vi "Scale Module (Main).vi"(7 "Name of Parent Panel":string="Main.vi", 9 "New Center Coords":T1={"Horizontal"=470, "Vertical"=200}, 10 "Config":variant, 11 "Main UI Message Queue":refnum<queue>) -> ()   [LabVIEW 2018, in "Scale Module.lvlib"]
doc: "This Continuous Measurement sample project is based on the Queued Message Handler template.\n\nThe Event Handling Loop generates messages based on user interface actions.\n\nThe Message Handling Loop processes messages generated by the Event Handling Loop, or by other messages. There are also Acquisition and Logging message handling loop subVIs, and a chart updating loop."
uses:
  Scale Module.lvlib
  support/Message Queue/Message Cluster.ctl
  <vilib>/Utility/miscctls.llb/LVPoint32TypeDef.ctl
  controls/UI State.ctl
  Feed Module/Controls/Scale Module State Cluster.ctl
  Feed Module/Controls/Scale Module Config Cluster.ctl
  Feed Module/Controls/Scale Module Settings Cluster.ctl
  Mettler Toledo/Controls/Settings Cluster.ctl
  Feed Module/Controls/Scale Module Display.ctl
  support/Message Queue/Enqueue Message (Single).vi
  support/User Event - Stop/User Event - Stop.lvlib
  support/Message Queue/Message Queue.lvlib
  support/Support Library.lvlib
  Measure Instrument/Scale Module Engine.lvlib
  Mettler Toledo/Mettler Toledo.lvlib
  Scale Settings Dialog.vi
  support/Command Log VIs/Command Logging.lvlib
  Report Generation/Report Generation.lvlib
panel:
  in  "Settings Button":bool
  out "Display Cluster":cluster{"User Name":string, "g":dbl} {"g" format="%#_5f"}
  out "H/W":dbl
  out "Original Height":u32
  out "Original Width":u32
  out "ScanCode":i16
  out "Log File path":path
  out "Status":string
  in  "Exit":bool
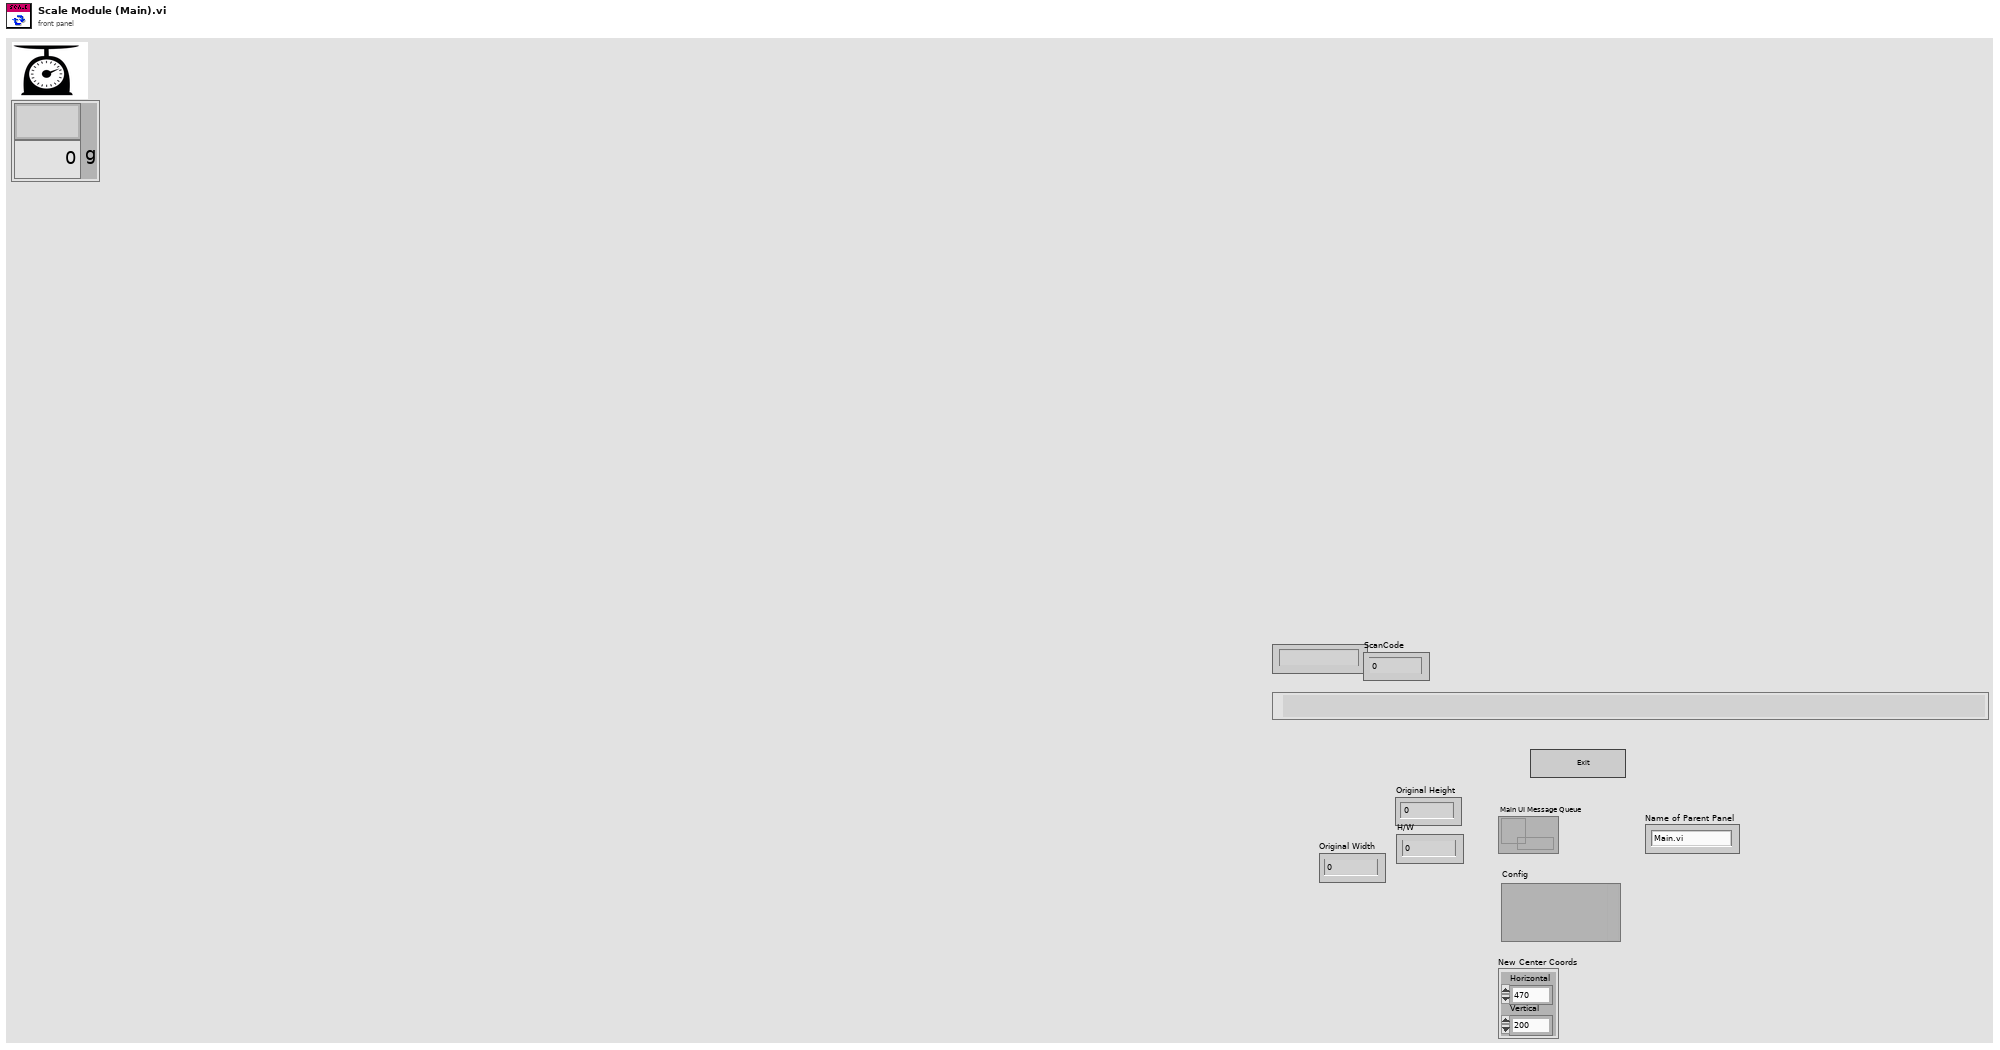
[diagram p1: front panel]
types:
  T1 = typedef "LVPoint32TypeDef.ctl" = cluster{"Horizontal":i32, "Vertical":i32}
  T2 = enum32{"Invalid", "Default", "Floating", "Floating/Auto-Hide", "Modal"}
  T3 = typedef "Scale Module.lvlib/Scale Module Config Cluster.ctl" = cluster{"GUID":string, "Drop Coords":T1, "Process Name":string, "User name":string, "Queue Name":string, "Settings":T4, "Load Count":i32}
  T4 = typedef "Scale Module.lvlib/Scale Module Settings Cluster.ctl" = cluster{"Cycle Period":dbl, "Mettler":T5, "Scale Type":string}
  T5 = typedef "Mettler Toledo.lvlib/Settings Cluster.ctl" = cluster{"VISA resource name":refnum<visa-resource-name>, "Simulated?":bool}
  T6 = typedef "UI State.ctl" = enum16{"Idle", "Acquiring and Logging", "Waiting for Exit", "Waiting for Exit (Acq Stopped)", "Waiting for Exit (Log Stopped)", "Waiting for Stop", "Waiting for Stop (Acq Stopped)", "Waiting for Stop (Log Stopped)"}
  T7 = typedef "Scale Module.lvlib/Scale Module State Cluster.ctl" = cluster{"Scale Module Config":T3}
  T8 = typedef "LVPointTypeDef.ctl" = cluster{"Horizontal":i16, "Vertical":i16}
  T9 = typedef "Scale Module.lvlib/Scale Message Queues.ctl" = cluster{"Scale UI":refnum<queue>, "Scale Engine":refnum<queue>, "Scale Display":refnum<queue>}
  T10 = typedef "Scale Module.lvlib/Scale Module Display.ctl" = cluster{"Scale Value":dbl, "Cycle Period":dbl}
  T11 = typedef "LVRectTypeDef.ctl" = cluster{"Left":i16, "Top":i16, "Right":i16, "Bottom":i16}
  T12 = cluster{"Shift":bool, "Ctrl":bool, "Alt":bool, "Cmd":bool, "Opt":bool}
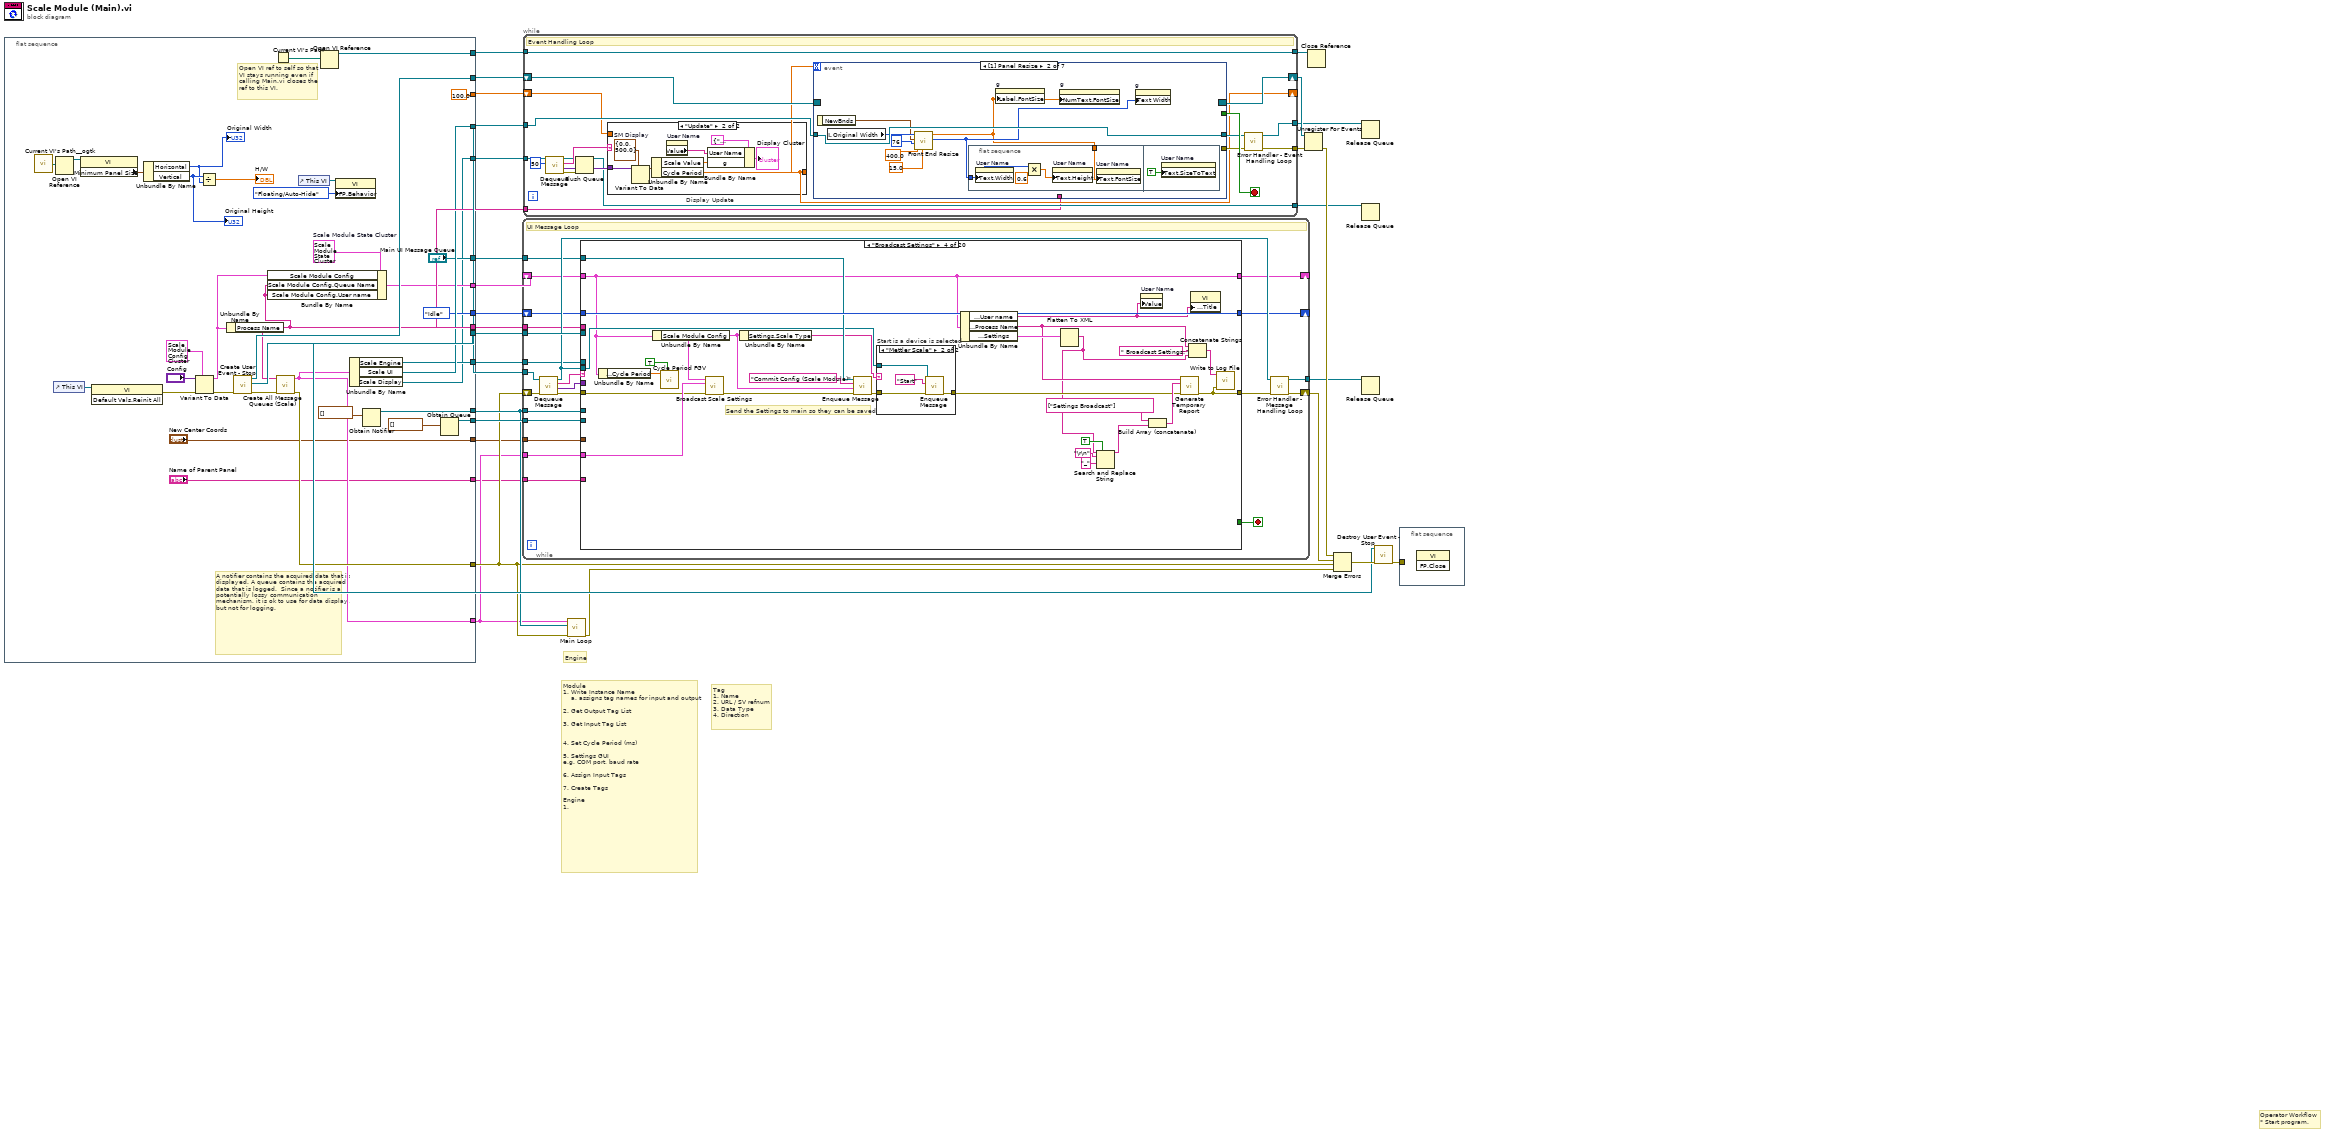
[diagram p0: block diagram]
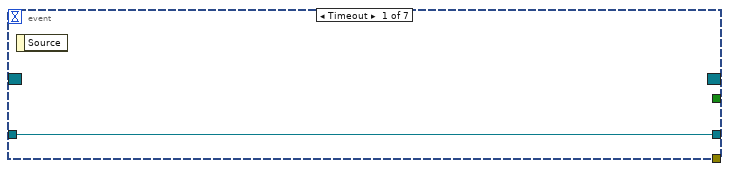
[diagram p3: hidden frame]
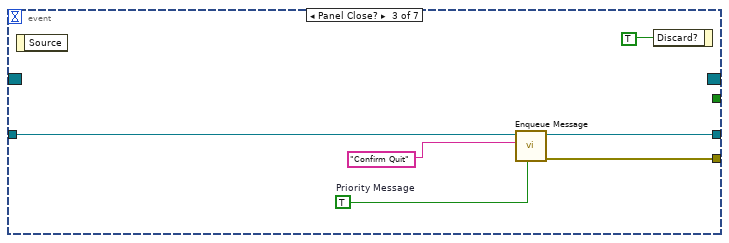
[diagram p4: hidden frame]
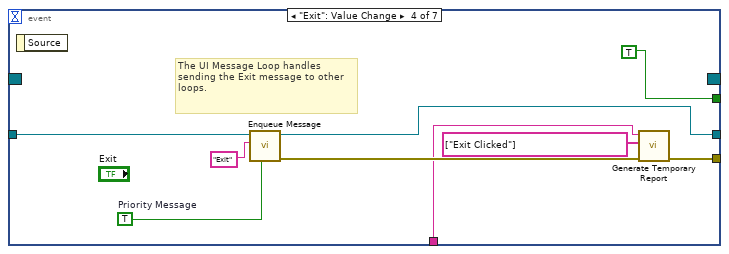
[diagram p5: hidden frame]
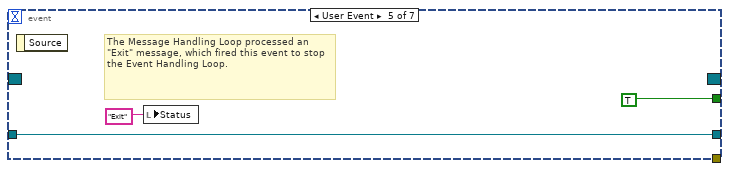
[diagram p6: hidden frame]
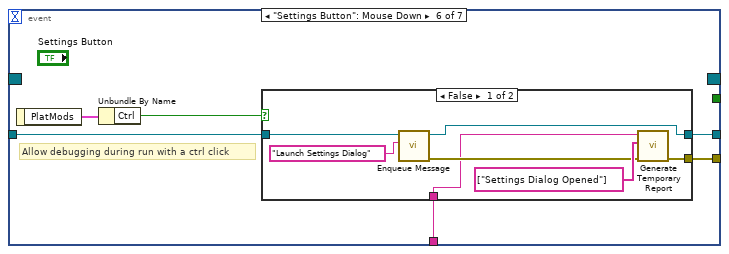
[diagram p7: hidden frame]
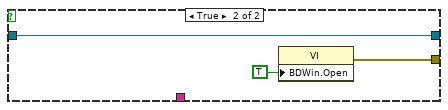
[diagram p8: hidden frame]
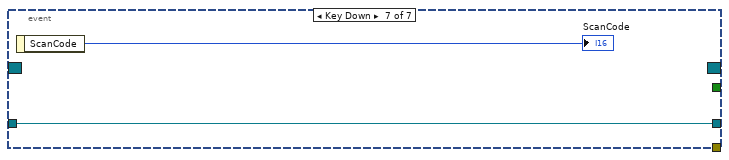
[diagram p9: hidden frame]
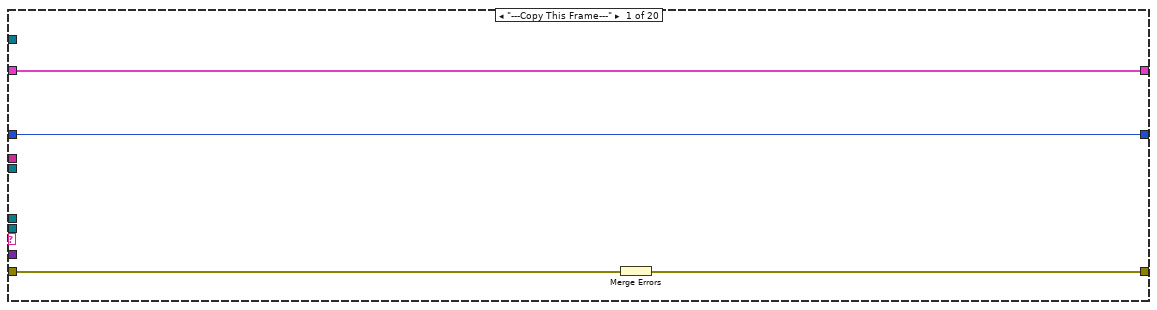
[diagram p10: hidden frame]
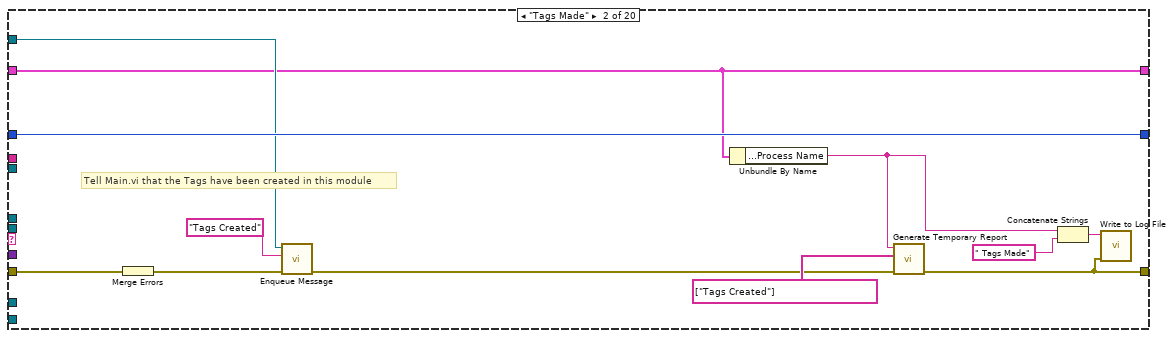
[diagram p11: hidden frame]
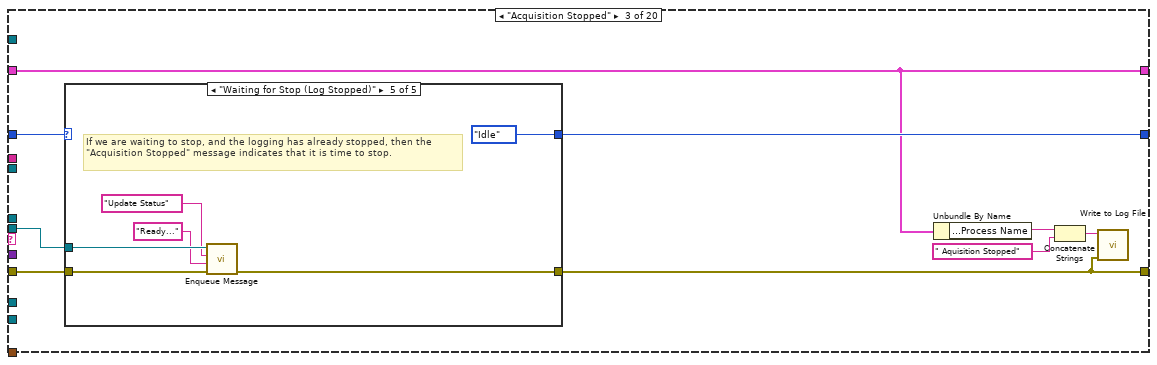
[diagram p12: hidden frame]
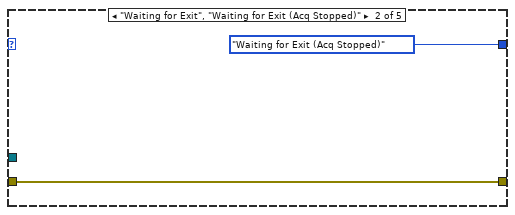
[diagram p14: hidden frame]
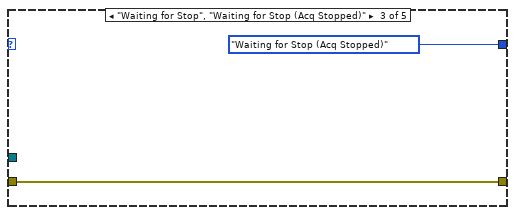
[diagram p15: hidden frame]
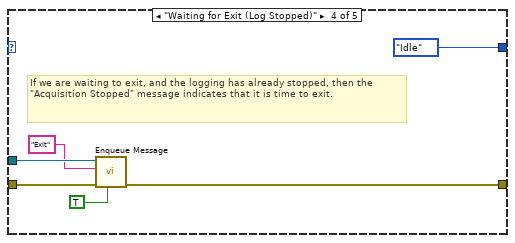
[diagram p16: hidden frame]
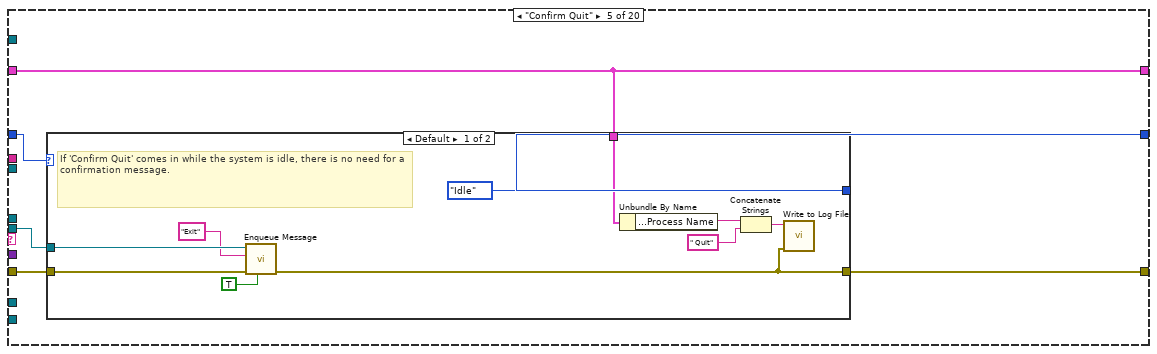
[diagram p18: hidden frame]
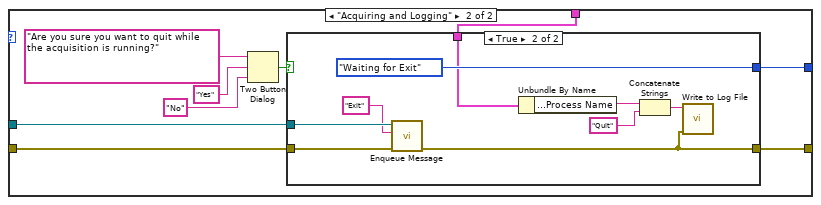
[diagram p19: hidden frame]
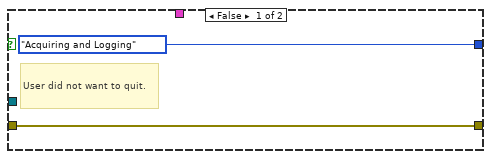
[diagram p20: hidden frame]
diagram:
  # "Engine"
  # "Operator Workflow\n* Start program."
  # "Module \n1. Write Instance Name\n    a. assigns tag names for input and output\n\n2. Get Output Tag List\n\n3. Get Input Tag List\n\n\n4. Set Cycle Period (ms)\n\n5. Settings GUI\ne.g. COM port, baud rate\n\n6. Assign Input Tags\n\n7. Create Tags\n\nEngine\n1."
  # "Tag\n1. Name\n2. URL / SV refnum\n3. Data Type\n4. Direction"
  n1 = flat-sequence {
    tunnel: [w64] -> w25
    tunnel: [w63] -> w24
    tunnel: [w62] -> w21
    tunnel: [UI_State."Idle" ("UI State")] -> w20
    tunnel: [w58] -> w19
    tunnel: [w57] -> w18
    tunnel: [w56] -> w16
    tunnel: [w55] -> w14
    tunnel: [w53] -> w13
    tunnel: ["Main UI Message Queue"] -> w12
    tunnel: [w48] -> w11
    tunnel: [w43] -> w10
    tunnel: [w42] -> w9
    tunnel: ["New Center Coords"] -> w8
    tunnel: ["Name of Parent Panel"] -> w7
    tunnel: [100.0 ("Cycle Period")] -> w5
    tunnel: [w35] -> w1
    frame #0 {
      w49 = T7 {"Scale Module Config"={"GUID"="PID1-Mettler Toledo Scale 1", "Drop Coords"={"Horizontal"=0, "Vertical"=0}, "Process Name"="PID1-Setpoint", "User name"="", "Queue Name"="", "Settings"={"Cycle Period"=500.0, "Mettler"={"VISA resource name"="", "Simulated?"=FALSE}, "Scale Type"=""}, "Load Count"=0}}  # Scale Module State Cluster
      # "Open VI ref to self so that\nVI stays running even if\ncalling Main.vi closes the\nref to this VI."
      # "A notifier contains the acquired data that is displayed. A queue contains the acquired data that is logged.  Since a notifier is a potentially lossy communication mechanism, it is ok to use for data display, but not for logging."
      n2 = call <userlib>:"Current VI's Path__ogtk.vi"() -> ("Current VI's Path (+ Relative)"=w30:path)  [unwired: 1 in]
      n3 = control-ref of="This VI"() -> (w46:refnum<vi>)
      n4 = Open VI Reference(vi path=w30) -> (vi reference=w31:refnum<vi>)  [unwired: 5 in, 1 out]
      n5 = property class="VI"(reference=w31) -> ("Minimum Panel Size"=w32:T8)  [unwired: 1 in, 2 out]
      n6 = invoke class="VI" method="Default Vals.Reinit All"(reference=w46) -> (error out=w39:errorcluster)  [unwired: 2 in, 2 out]
      n7 = Unbundle By Name(w32) -> ("Horizontal"=w33:i16, "Vertical"=w34:i16)
      "Original Width" <- w33
      "Original Height" <- w34
      n8 = Variant To Data(error in=w39, type=T3 {"GUID"="", "Drop Coords"={"Horizontal"=0, "Vertical"=0}, "Process Name"="", "User name"="", "Queue Name"="", "Settings"={"Cycle Period"=500.0, "Mettler"={"VISA resource name"="", "Simulated?"=FALSE}, "Scale Type"=""}, "Load Count"=0} ("Feed Module Config"), Variant="Config") -> (data=w47:T3, error out=w52:errorcluster)
      n9 = Divide(x=w34, y=w33) -> (x/y=→"H/W":dbl)
      n10 = Unbundle By Name(w47) -> ("Process Name"=w35:string)
      n11 = call "Create User Event - Stop.vi"("error in (no error)"=w52) -> ("error out"=w44:errorcluster, "User Event - Stop"=w63:refnum<user-event>, "Stop Event Registration Refnum"=w64:refnum<event-registration>)  [unwired: 8 in]
      n12 = Bundle By Name(cluster=w49, "Scale Module Config"=w47, "Scale Module Config.Queue Name"=w35, "Scale Module Config.User name"=w35) -> (w53:T7)
      n13 = Current VI's Path() -> (path=w54:path)
      n14 = call "Create All Message Queues (Scale).vi"("error in (no error)"=w44, "Process Name"=w35) -> ("error out"=w43:errorcluster, "Message Queues"=w42:T9)  [unwired: 8 in]
      n15 = control-ref of="This VI"() -> (w37:refnum<vi>)
      n16 = Open VI Reference(vi path=w54) -> (vi reference=w55:refnum<vi>)  [unwired: 5 in, 1 out]
      n17 = property class="VI"(reference=w37, "FP.Behavior"=T2."Floating/Auto-Hide" ("Front Panel Window:Behavior")) -> ()  [unwired: 1 in, 2 out]
      n18 = Unbundle By Name(w42) -> ("Scale Engine"=w58:refnum<queue>, "Scale UI"=w62:refnum<queue>, "Scale Display"=w48:refnum<queue>)
      n19 = Obtain Notifier(notification data type=waveform(dbl)[] []) -> (notifier out=w56:refnum<notifier>)  [unwired: 3 in, 2 out]
      n20 = Obtain Queue(element data type=waveform(dbl)[] []) -> (queue out=w57:refnum<queue>)  [unwired: 4 in, 2 out]
    }
  }
  n21 = while {
    tunnel: w21 -> [w82]
    tunnel: w24 -> [w86]
    shift-right: [w78] -> w28
    shift-left: w10 -> [w85]
    shift-right: [w69] -> _
    shift-left: w13 -> [w71]
    tunnel: w16 -> [w81]
    tunnel: w18 -> [w80]
    shift-right: [w75] -> _
    shift-left: w20 -> [w76]
    tunnel: w19 -> [w74]
    tunnel: w9 -> [w73]
    tunnel: w12 -> [w70]
    tunnel: w1 -> [w68]
    tunnel: w8 -> [w67]
    tunnel: w7 -> [w66]
    tunnel: [w65] -> w2
    stop <- w87 stop-if-true
    # "UI Message Loop"
    n22 = call "Dequeue Message.vi"("error in (no error)"=w85, "Message Queue"=w82) -> ("error out"=w72:errorcluster, "Message Data"=w83:variant, "Message"=w84:string, "dup Message Queue"=w77:refnum<queue>)  [unwired: 6 in]
    n23 = case "Message Cases" shown="\"Broadcast Settings\"" w84 {
      selector: w84 -> [_ _ _ _ _ _ _ _ _ _ _ _ _ _ _ _ _ _ _ w435]
      tunnel: w77 -> [_ _ w109 w149 w167 _ w219 w233 w257 _ w298 w314 w334 _ w372 _ _ w423 _ _]
      tunnel: w72 -> [w91 w103 w110 w153 w166 w201 w214 w237 w256 w282 w294 w313 w335 w359 w371 w380 w391 w418 w432 _]
      tunnel: [w90 w92 w105 w135 w165 w202 w206 w224 w238 w282 w284 w307 w330 w362 w367 w376 w393 w407 w433 w434] -> w79
      tunnel: [_ _ _ _ _ _ _ _ TRUE _ _ _ _ _ _ _ _ _ _ _] -> w87
      tunnel: w83 -> [_ _ _ _ _ w204 _ w236 w246 _ _ _ _ w360 _ _ _ _ w431 _]
      tunnel: w86 -> [_ _ _ _ _ _ _ _ w267 _ _ _ _ _ _ _ _ _ _ _]
      tunnel: w71 -> [w88 w96 w104 w143 w163 w199 w210 w223 w242 w279 w287 w306 w329 w365 w366 w381 w392 w411 w426 w440]
      tunnel: w81 -> [_ _ _ _ _ _ _ _ w265 _ _ _ _ _ _ _ _ _ _ _]
      tunnel: w80 -> [_ _ _ _ _ _ _ _ w261 _ _ _ _ _ _ _ _ _ _ _]
      tunnel: w76 -> [w89 w102 w112 w157 w168 w200 w215 w228 w254 _ _ w315 w337 w364 _ _ _ w419 w427 w444]
      tunnel: [w89 w102 w111 w157 w164 w200 w216 w228 w253 UI_State."Idle" ("UI State") UI_State."Idle" ("UI State") w315 w336 w364 UI_State."Acquiring and Logging" ("UI State") UI_State."Acquiring and Logging" ("UI State") UI_State."Acquiring and Logging" ("UI State") w420 w427 w444] -> w75
      tunnel: w74 -> [_ _ _ _ _ _ _ _ w260 _ _ _ _ _ _ w384 w400 w417 _ _]
      tunnel: w73 -> [_ _ _ w156 _ _ _ _ _ _ _ _ _ _ _ _ _ _ _ _]
      tunnel: w70 -> [_ w99 _ w150 _ _ _ _ w245 _ _ _ _ _ _ _ _ _ _ _]
      tunnel: [w88 w96 w104 w143 w163 w199 w210 w223 w242 w279 w287 w305 w329 w365 w366 w381 w392 w411 w426 w440] -> w69
      tunnel: w68 -> [_ _ _ _ _ _ _ _ _ _ w292 _ _ _ _ _ _ _ _ _]
      tunnel: w67 -> [_ _ _ _ _ _ _ _ _ _ w291 _ _ _ _ _ _ _ _ _]
      tunnel: w66 -> [_ _ _ _ _ _ _ _ _ _ w290 _ _ _ _ _ _ _ _ _]
      frame "---Copy This Frame---" {
        # "Duplicate this frame when creating new messages.  Change this comment in the duplicated frame to describe this message."
        n24 = Merge Errors(w91) -> (w90:errorcluster)
      }
      frame "Tags Made" {
        # "Tell Main.vi that the Tags have been created in this module"
        # "Duplicate this frame when creating new messages.  Change this comment in the duplicated frame to describe this message."
        n25 = Merge Errors(w103) -> (w100:errorcluster)
        n26 = call-poly "Enqueue Message.vi"("error in (no error)"=w100, "Message"="Tags Created", "Message Queue"=w99) -> ("error out"=w93:errorcluster)  [unwired: 7 in, 1 out]
        n27 = Unbundle By Name(w96) -> ("Scale Module Config.Process Name"=w94:string)
        n28 = call "Generate Temporary Report.vi"("error in (no error)"=w93, "Line of Events"=string[] ["Tags Created"], "Module Name"=w94) -> ("error out"=w92:errorcluster)  [unwired: 8 in]
        n29 = Concatenate Strings(w94, " Tags Made" ("text")) -> (w97:string)
        n30 = call "Write to Log File.vi"("error in"=w92, "text"=w97) -> ()  [unwired: 9 in, 1 out]
      }
      frame "Acquisition Stopped" {
        # "Logic for determining what action to take when the acquisition has stopped."
        n31 = case shown="\"Waiting for Stop (Log Stopped)\"" w112 {
          selector: w112 -> [w114 _ _ _ _]
          tunnel: [w114 UI_State."Waiting for Exit (Acq Stopped)" ("UI State") UI_State."Waiting for Stop (Acq Stopped)" ("UI State") UI_State."Idle" ("UI State") UI_State."Idle" ("UI State")] -> w111
          tunnel: w110 -> [w113 w115 w117 w123 w129]
          tunnel: [w113 w115 w117 w122 w128] -> w105
          tunnel: w109 -> [_ _ _ w121 w127]
          frame Default {
          }
          frame "Waiting for Exit", "Waiting for Exit (Acq Stopped)" {
          }
          frame "Waiting for Stop", "Waiting for Stop (Acq Stopped)" {
          }
          frame "Waiting for Exit (Log Stopped)" {
            # "If we are waiting to exit, and the logging has already stopped, then the \"Acquisition Stopped\" message indicates that it is time to exit."
            n32 = call-poly "Enqueue Message.vi"("Priority Message? (F)"=TRUE, "error in (no error)"=w123, "Message"="Exit", "Message Queue"=w121) -> ("error out"=w122:errorcluster)  [unwired: 6 in, 1 out]
          }
          frame "Waiting for Stop (Log Stopped)" {
            # "If we are waiting to stop, and the logging has already stopped, then the \"Acquisition Stopped\" message indicates that it is time to stop."
            n33 = call-poly "Enqueue Message.vi"("error in (no error)"=w129, "Message Data"="Ready..." ("Message"), "Message"="Update Status", "Message Queue"=w127) -> ("error out"=w128:errorcluster)  [unwired: 6 in, 1 out]
          }
        }
        n34 = Unbundle By Name(w104) -> ("Scale Module Config.Process Name"=w108:string)
        n35 = Concatenate Strings(w108, " Aquisition Stopped" ("text")) -> (w106:string)
        n36 = call "Write to Log File.vi"("error in"=w105, "text"=w106) -> ()  [unwired: 9 in, 1 out]
      }
      frame "Broadcast Settings" {
        # "Send the Settings to main so they can be saved"
        # "Send the 'Update Settings' message to the Logging and Acquisition message loops."
        n37 = Unbundle By Name(w143) -> ("Scale Module Config.Settings.Cycle Period"=w154:dbl)
        n38 = Unbundle By Name(w143) -> ("Scale Module Config"=w146:T3)
        n39 = call "Cycle Period FGV.vi"("Write"=TRUE, "Cycle Period In (ms)"=w154) -> ()  [unwired: 8 in, 2 out]
        n40 = call "Broadcast Scale Settings.vi"("error in (no error)"=w153, "Message Queues"=w156, "Scale Module Config"=w146) -> ("error out"=w151:errorcluster)  [unwired: 8 in]
        n41 = Unbundle By Name(w146) -> ("Settings.Scale Type"=w147:string)
        n42 = call-poly "Enqueue Message.vi"("error in (no error)"=w151, "Message Data"=w146, "Message"="Commit Config (Scale Module)", "Message Queue"=w150) -> ("error out"=w148:errorcluster)  [unwired: 6 in, 1 out]
        n43 = case "Start is a device is selected" shown="\"Mettler Scale\"" w147 {
          tunnel: w149 -> [_ w161]
          tunnel: w148 -> [w158 w160]
          tunnel: [w158 w159] -> w136
          frame "False", Default {
          }
          frame "Mettler Scale" {
            n44 = call-poly "Enqueue Message.vi"("error in (no error)"=w160, "Message"="Start", "Message Queue"=w161) -> ("error out"=w159:errorcluster)  [unwired: 7 in, 1 out]
          }
        }
        n45 = Unbundle By Name(w143) -> ("Scale Module Config.User name"=w131:string, "Scale Module Config.Process Name"=w134:string, "Scale Module Config.Settings"=w142:T4)
        n46 = Flatten To XML(anything=w142) -> (xml string=w133:string)
        n47 = Search and Replace String(replace all?=TRUE ("replace all? (F)"), input string=w133, search string="\r\n", replace string="_" ("replace string (\"\")")) -> (result string=w132:string)  [unwired: 4 in, 3 out]
        n48 = property on="User Name" class="Str"("Value"=w131) -> ()  [unwired: 2 in, 2 out]
        n49 = Build Array (concatenate)(string[] ["Settings Broadcast"] ("Line of Events"), w132) -> (w137:string[])
        n50 = call "Generate Temporary Report.vi"("error in (no error)"=w136, "Line of Events"=w137, "Module Name"=w134) -> ("error out"=w135:errorcluster)  [unwired: 8 in]
        n51 = Concatenate Strings(w134, " Broadcast Settings: " ("text"), w133) -> (w144:string)
        n52 = property class="VI"("Front Panel.Title"=w131) -> ()  [unwired: 2 in, 2 out]
        n53 = call "Write to Log File.vi"("error in"=w135, "text"=w144) -> ()  [unwired: 9 in, 1 out]
      }
      frame "Confirm Quit" {
        # "Confirm Quit - Message that can confirm whether or not the user wants to exit the application."
        n54 = case shown="Default" w168 {
          tunnel: w167 -> [w177 w184]
          tunnel: w166 -> [w176 w182]
          tunnel: [w170 w181] -> w165
          tunnel: [UI_State."Idle" ("UI State") w180] -> w164
          tunnel: w163 -> [w169 w179]
          frame Default {
            # "If 'Confirm Quit' comes in while the system is idle, there is no need for a confirmation message."
            n55 = call-poly "Enqueue Message.vi"("Priority Message? (F)"=TRUE, "error in (no error)"=w176, "Message"="Exit", "Message Queue"=w177) -> ("error out"=w170:errorcluster)  [unwired: 6 in, 1 out]
            n56 = Unbundle By Name(w169) -> ("Scale Module Config.Process Name"=w173:string)
            n57 = Concatenate Strings(w173, " Quit" ("text")) -> (w171:string)
            n58 = call "Write to Log File.vi"("error in"=w170, "text"=w171) -> ()  [unwired: 9 in, 1 out]
          }
          frame "Acquiring and Logging" {
            n59 = Two Button Dialog(message="Are you sure you want to quit while the acquisition is running?" ("Confirm Quit Message"), 1:"No" ("No"), 2:"Yes" ("Yes")) -> (T button?=w183:bool)
            n60 = case shown="True" w183 {
              tunnel: w184 -> [_ w198]
              tunnel: w182 -> [w188 w197]
              tunnel: [w188 w191] -> w181
              tunnel: [UI_State."Acquiring and Logging" ("UI State") UI_State."Waiting for Exit" ("UI State")] -> w180
              tunnel: w179 -> [_ w190]
              frame False {
                # "User did not want to quit."
              }
              frame True {
                n61 = call-poly "Enqueue Message.vi"("error in (no error)"=w197, "Message"="Exit", "Message Queue"=w198) -> ("error out"=w191:errorcluster)  [unwired: 7 in, 1 out]
                n62 = Unbundle By Name(w190) -> ("Scale Module Config.Process Name"=w194:string)
                n63 = Concatenate Strings(w194, "Quit" ("text")) -> (w192:string)
                n64 = call "Write to Log File.vi"("error in"=w191, "text"=w192) -> ()  [unwired: 9 in, 1 out]
              }
            }
          }
        }
      }
      frame "Display Log File Path" {
        n65 = Variant To Data(error in=w201, type=path "", Variant=w204) -> (data=→"Log File path":path, error out=w202:errorcluster)
      }
      frame "E-Stop" {
        # "E-Stop has no effect on the scale"
        # "Message Acquisition and Logging loops to stop"
        # "Stop the pumps."
        n66 = call-poly "Enqueue Message.vi"("error in (no error)"=w214, "Message Data"="Ready..." ("Ready..."), "Message"="Update Status", "Message Queue"=w219) -> ("error out"=w213:errorcluster)  [unwired: 6 in, 1 out]
        n67 = case shown="\"Waiting for Exit\"" w215 {
          selector: w215 -> [_ w221]
          tunnel: [UI_State."Waiting for Stop" ("UI State") w221] -> w216
          frame Default {
          }
          frame "Waiting for Exit" {
          }
        }
        n68 = Merge Errors(w213) -> (w207:errorcluster)
        n69 = Unbundle By Name(w210) -> ("Scale Module Config.Process Name"=w208:string)
        n70 = call "Generate Temporary Report.vi"("error in (no error)"=w207, "Line of Events"=string[] ["E-STOP"], "Module Name"=w208) -> ("error out"=w206:errorcluster)  [unwired: 8 in]
        n71 = Concatenate Strings(w208, " E-STOP" ("text")) -> (w211:string)
        n72 = call "Write to Log File.vi"("error in"=w206, "text"=w211) -> ()  [unwired: 9 in, 1 out]
      }
      frame "Error" {
        # "Error - Check the error message data and respond accordingly. This message is sent by the \"Error Handler\" VIs at the end of each loop in this application."
        n73 = Variant To Data(error in=w237, type=errorcluster {"status"=FALSE, "code"=0, "source"=""} ("error out"), Variant=w236) -> (data=w234:errorcluster, error out=w230:errorcluster)
        n74 = call <vilib>:"General Error Handler.vi"("error in (no error)"=w234) -> ("message"=w222:string)  [unwired: 10 in, 4 out]
        n75 = call-poly "Enqueue Message.vi"("Priority Message? (F)"=TRUE, "Message"="Exit", "Message Queue"=w233) -> ("error out"=w229:errorcluster)  [unwired: 7 in, 1 out]
        n76 = Merge Errors(w229, w230) -> (w224:errorcluster)
        n77 = Unbundle By Name(w223) -> ("Scale Module Config.Process Name"=w227:string)
        n78 = Concatenate Strings(w227, " Error: " ("text"), w222) -> (w225:string)
        n79 = call "Write to Log File.vi"("error in"=w224, "text"=w225) -> ()  [unwired: 9 in, 1 out]
      }
      frame "Exit" {
        w249 = TRUE  # Delete Module?
        # "Don't check the error outs. The acquisition and logging queues may have already been released."
        # "Close references owned by the Main VI."
        # "Stop the VI"
        # "Exit - Fire the User Event to stop the Event Handling Loop.  Also send Exit messages to the Acquisition and Logging loops."
        n80 = call "Fire User Event - Stop.vi"("User Event - Stop"=w267) -> ("error out"=w266:errorcluster)  [unwired: 10 in]
        n81 = Build Array(w260) -> (w259:refnum<queue>[])
        n82 = for {
          tunnel: w259 -> [w276] mode=indexing
          n83 = call-poly "Enqueue Message.vi"("Message"="Stop", "Message Queue"=w276) -> ("dup Message Queue"=w277:refnum<queue>)  [unwired: 8 in, 1 out]
          n84 = call-poly "Enqueue Message.vi"("Message"="Exit", "Message Queue"=w277) -> ()  [unwired: 8 in, 2 out]
        }
        n85 = Variant To Data(type=w249, Variant=w246) -> (data=w248:bool, error out=w250:errorcluster)  [unwired: 1 in]
        n86 = call-poly "Enqueue Message.vi"("error in (no error)"=w256, "Message Data"="Ready..." ("Ready..."), "Message"="Update Status", "Message Queue"=w257) -> ("error out"=w255:errorcluster, "dup Message Queue"=w252:refnum<queue>)  [unwired: 6 in]
        n87 = Select(t=w249, s=w250, f=w248) -> (s? t:f=w247:bool)
        n88 = case "Don't enqueue Delete Module if opening campaign because it\nwill already have been deleted and new config loaded and we create\na race condition." shown="True" w247 {
          tunnel: w245 -> [_ w271]
          tunnel: w242 -> [_ w270]
          frame False {
          }
          frame True {
            n89 = Unbundle By Name(w270) -> ("Scale Module Config.GUID"=w269:string)
            n90 = call-poly "Enqueue Message.vi"("Message Data"=w269, "Message"="Delete Module", "Message Queue"=w271) -> ()  [unwired: 7 in, 2 out]
          }
        }
        n91 = Release Queue(queue=w252, error in (no error)=w255) -> (error out=w264:errorcluster)  [unwired: 1 in, 2 out]
        n92 = Release Notifier(notifier=w265, error in (no error)=w264) -> (error out=w263:errorcluster)  [unwired: 1 in, 2 out]
        n93 = case shown="Default" w254 {
          selector: w254 -> [_ w274]
          tunnel: [UI_State."Waiting for Stop" ("UI State") w274] -> w253
          frame Default {
          }
          frame "Waiting for Exit" {
          }
        }
        n94 = Release Queue(queue=w261, error in (no error)=w263) -> (error out=w262:errorcluster)  [unwired: 1 in, 2 out]
        n95 = Merge Errors(w266, w262) -> (w239:errorcluster)
        n96 = Unbundle By Name(w242) -> ("Scale Module Config.Process Name"=w240:string)
        n97 = Concatenate Strings(w240, " Exit" ("text")) -> (w243:string)
        n98 = call "Generate Temporary Report.vi"("error in (no error)"=w239, "Line of Events"=string[] ["Exited"], "Module Name"=w240) -> ("error out"=w238:errorcluster)  [unwired: 8 in]
        n99 = call "Write to Log File.vi"("error in"=w238, "text"=w243) -> ()  [unwired: 9 in, 1 out]
      }
      frame "Init UI Refs" {
        # "Init UI Refs - Store control references for UI controls.  Also enable/disable controls appropriately."
        n100 = property class="VI"("Front Panel.Closeable"=TRUE ("Front Panel Window:Closeable")) -> ()  [unwired: 2 in, 2 out]
      }
      frame "Initialize" {
        # "Initialize - Get configuration settings, then message the UI to initialize, and broadcast the settings to the other message loops."
        n101 = call-poly "Enqueue Message.vi"("error in (no error)"=w294, "Message"="Init UI Refs", "Message Queue"=w298) -> ("error out"=w296:errorcluster, "dup Message Queue"=w297:refnum<queue>)  [unwired: 7 in]
        n102 = property class="VI" props=["FP.State"]() -> (reference out=w293:refnum<vi>)  [unwired: 2 in, 2 out]
        n103 = call "Make Child and Move.vi"("Process Name"=w292, "Name of Parent Panel"=w290, "New Center Coords"=w291, "VI in"=w293) -> ()  [unwired: 8 in]
        n104 = call-poly "Enqueue Message.vi"("error in (no error)"=w296, "Message"="Broadcast Settings", "Message Queue"=w297) -> ("error out"=w304:errorcluster, "dup Message Queue"=w303:refnum<queue>)  [unwired: 7 in]
        n105 = call-poly "Enqueue Message.vi"("error in (no error)"=w304, "Message Data"="Ready..." ("Ready..."), "Message"="Update Status", "Message Queue"=w303) -> ("error out"=w285:errorcluster)  [unwired: 6 in, 1 out]
        n106 = Unbundle By Name(w287) -> ("Scale Module Config.Process Name"=w283:string)
        n107 = call "Generate Temporary Report.vi"("error in (no error)"=w285, "Line of Events"=string[] ["Initialized"], "Module Name"=w283) -> ("error out"=w284:errorcluster)  [unwired: 8 in]
        n108 = Concatenate Strings(w283, " Initialize" ("text")) -> (w288:string)
        n109 = call "Write to Log File.vi"("error in"=w284, "text"=w288) -> ()  [unwired: 9 in, 1 out]
      }
      frame "Launch Settings Dialog" {
        # "Launch the Settings Dialog when the user clicks the 'Settings' button."
        n110 = in-place {
          in-place-border: w313 -> [w321]
          in-place-border: [w320] -> w312
          in-place-border: [w319] -> w311
          n111 = in-place-cluster #1(w306) -> ("Scale Module Config"=w317:T3)
          n112 = in-place {
            n113 = in-place-cluster #2(w317) -> ("Load Count"=w322:i32)
            n114 = Increment(x=w322) -> (x+1=w323:i32)
            n115 = in-place-cluster #2("Load Count"=w323) -> (w318:T3)
          }
          n116 = call-by-ref "?"("error in (no error)"=w321, "Scale Module Config In"=w318) -> ("error out"=w320:errorcluster, "Cancelled?"=w319:bool, "Scale Module Config Out"=w316:T3)  [unwired: 8 in, 3 out]
          n117 = in-place-cluster #1("Scale Module Config"=w316) -> (w305:T7)
        }
        n118 = case shown="False" w311 {
          tunnel: w312 -> [w325 w328]
          tunnel: [w324 w328] -> w307
          tunnel: w314 -> [w327 _]
          frame False {
            n119 = call-poly "Enqueue Message.vi"("error in (no error)"=w325, "Message"="Broadcast Settings", "Message Queue"=w327) -> ("error out"=w324:errorcluster)  [unwired: 7 in, 1 out]
          }
          frame True {
          }
        }
        n120 = Unbundle By Name(w305) -> ("Scale Module Config.Process Name"=w310:string)
        n121 = Concatenate Strings(w310, " Setting Dialog Launched" ("text")) -> (w308:string)
        n122 = call "Write to Log File.vi"("error in"=w307, "text"=w308) -> ()  [unwired: 9 in, 1 out]
      }
      frame "Logging Stopped" {
        # "Logic for determining what action to take when the logging has stopped."
        n123 = case shown="\"Waiting for Exit (Acq Stopped)\"" w337 {
          selector: w337 -> [w339 _ _ _ _]
          tunnel: [w339 UI_State."Waiting for Exit (Log Stopped)" ("UI State") UI_State."Waiting for Stop (Log Stopped)" ("UI State") UI_State."Idle" ("UI State") UI_State."Idle" ("UI State")] -> w336
          tunnel: w335 -> [w338 w340 w342 w348 w354]
          tunnel: [w338 w340 w342 w347 w353] -> w330
          tunnel: w334 -> [_ _ _ w346 w352]
          frame Default {
          }
          frame "Waiting for Exit", "Waiting for Exit (Log Stopped)" {
          }
          frame "Waiting for Stop", "Waiting for Stop (Log Stopped)" {
          }
          frame "Waiting for Exit (Acq Stopped)" {
            # "If we are waiting to exit, and the acquisition has already stopped, then the \"Logging Stopped\" message indicates that it is time to exit."
            n124 = call-poly "Enqueue Message.vi"("Priority Message? (F)"=TRUE, "error in (no error)"=w348, "Message"="Exit", "Message Queue"=w346) -> ("error out"=w347:errorcluster)  [unwired: 6 in, 1 out]
          }
          frame "Waiting for Stop (Acq Stopped)" {
            # "If we are waiting to stop, and the acquisition has already stopped, then the \"Logging Stopped\" message indicates that it is time to stop."
            n125 = call-poly "Enqueue Message.vi"("error in (no error)"=w354, "Message Data"="Ready..." ("Message"), "Message"="Update Status", "Message Queue"=w352) -> ("error out"=w353:errorcluster)  [unwired: 6 in, 1 out]
          }
        }
        n126 = Unbundle By Name(w329) -> ("Scale Module Config.Process Name"=w333:string)
        n127 = Concatenate Strings(w333, " Logging Stopped" ("text")) -> (w331:string)
        n128 = call "Write to Log File.vi"("error in"=w330, "text"=w331) -> ()  [unwired: 9 in, 1 out]
      }
      frame "Send to Sequence" {
        n129 = Variant To Data(error in=w359, type=refnum<queue> refnum ("Message Queue"), Variant=w360) -> (data=w357:refnum<queue>, error out=w358:errorcluster)
        n130 = property on="g" class="DigNum (strict)"() -> ("Value"=w356:dbl)  [unwired: 2 in, 2 out]
        n131 = call-poly "Enqueue Message.vi"("error in (no error)"=w358, "Message Data"=w356, "Message"="Sent to Sequence", "Message Queue"=w357) -> ("error out"=w362:errorcluster)  [unwired: 6 in, 1 out]
      }
      frame "Start" {
        # "Message Acquisition and Logging loops to start"
        # "Start - Enable/Disable buttons appropriately for an acquisition that has started, and update status display."
        n132 = call-poly "Enqueue Message.vi"("error in (no error)"=w371, "Message"="Start Loops", "Message Queue"=w372) -> ("error out"=w373:errorcluster)  [unwired: 7 in, 1 out]
        n133 = Merge Errors(w373) -> (w367:errorcluster)
        n134 = Unbundle By Name(w366) -> ("Scale Module Config.Process Name"=w370:string)
        n135 = Concatenate Strings(w370, " Start" ("text")) -> (w368:string)
        n136 = call "Write to Log File.vi"("error in"=w367, "text"=w368) -> ()  [unwired: 9 in, 1 out]
      }
      frame "Start Loops" {
        # "I'm not sure what we would have multiple Process names in a module for but i'll leave it for now."
        # "Message Acquisition and Logging loops to start"
        # "Start - Enable/Disable buttons appropriately for an acquisition that has started, and update status display."
        n137 = Unbundle By Name(w381) -> ("Scale Module Config.Process Name"=w377:string)
        n138 = Build Array(w384) -> (w382:refnum<queue>[])
        n139 = for {
          tunnel: w380 -> [w389]
          tunnel: [w388] -> w383 mode=indexing
          tunnel: w382 -> [w387] mode=indexing
          tunnel: w377 -> [w386]
          n140 = call-poly "Enqueue Message.vi"("error in (no error)"=w389, "Message Data"=w386, "Message"="Start", "Message Queue"=w387) -> ("error out"=w388:errorcluster)  [unwired: 6 in, 1 out]
        }
        n141 = Merge Errors(w380, w383) -> (w378:errorcluster)
        n142 = call "Generate Temporary Report.vi"("error in (no error)"=w378, "Line of Events"=string[] ["Started"], "Module Name"=w377) -> ("error out"=w376:errorcluster)  [unwired: 8 in]
      }
      frame "Start Log" {
        # "I'm not sure what we would have multiple Process names in a module for but i'll leave it for now."
        # "Message Acquisition and Logging loops to start"
        # "Start - Enable/Disable buttons appropriately for an acquisition that has started, and update status display."
        n143 = Unbundle By Name(w392) -> ("Scale Module Config.Process Name"=w397:string)
        n144 = Build Array(w400) -> (w398:refnum<queue>[])
        n145 = for {
          tunnel: w391 -> [w405]
          tunnel: [w404] -> w399 mode=indexing
          tunnel: w398 -> [w403] mode=indexing
          tunnel: w397 -> [w402]
          n146 = call-poly "Enqueue Message.vi"("error in (no error)"=w405, "Message Data"=w402, "Message"="Start Log", "Message Queue"=w403) -> ("error out"=w404:errorcluster)  [unwired: 6 in, 1 out]
        }
        n147 = Merge Errors(w391, w399) -> (w393:errorcluster)
        n148 = Unbundle By Name(w392) -> ("Scale Module Config.Process Name"=w396:string)
        n149 = Concatenate Strings(w396, " Start Log" ("text")) -> (w394:string)
        n150 = call "Write to Log File.vi"("error in"=w393, "text"=w394) -> ()  [unwired: 9 in, 1 out]
      }
      frame "Stop" {
        # "Stop - Enable/Disable buttons appropriately for an acquisition that has stopped, and update status display."
        n151 = call-poly "Enqueue Message.vi"("error in (no error)"=w418, "Message Data"="Ready..." ("Ready..."), "Message"="Update Status", "Message Queue"=w423) -> ("error out"=w416:errorcluster)  [unwired: 6 in, 1 out]
        n152 = call-poly "Enqueue Message.vi"("error in (no error)"=w416, "Message"="Stop", "Message Queue"=w417) -> ("error out"=w414:errorcluster)  [unwired: 7 in, 1 out]
        n153 = case shown="Default" w419 {
          selector: w419 -> [_ w425]
          tunnel: [UI_State."Waiting for Stop" ("UI State") w425] -> w420
          frame Default {
          }
          frame "Waiting for Exit" {
          }
        }
        n154 = Merge Errors(w414) -> (w408:errorcluster)
        n155 = Unbundle By Name(w411) -> ("Scale Module Config.Process Name"=w409:string)
        n156 = Concatenate Strings(w409, " Stop" ("text")) -> (w412:string)
        n157 = call "Generate Temporary Report.vi"("error in (no error)"=w408, "Line of Events"=string[] ["Stopped"], "Module Name"=w409) -> ("error out"=w407:errorcluster)  [unwired: 8 in]
        n158 = call "Write to Log File.vi"("error in"=w407, "text"=w412) -> ()  [unwired: 9 in, 1 out]
      }
      frame "Update Status" {
        # "Update Display - Convert the message data to a string to display in the Status indicator."
        n159 = Variant To Data(error in=w432, type="", Variant=w431) -> (data=→"Status":string, error out=w429:errorcluster)
        n160 = Merge Errors(w429) -> (w433:errorcluster)
      }
      frame Default {
        # "'Default' case only runs if there is a message that isn't defined in any of the other cases.  Output a programming error."
        n161 = Concatenate Strings("The invalid message string " ("string"), w435, " was received in Scale Module Main" ("string")) -> (w436:string)
        n162 = Bundle By Name(cluster=errorcluster {"status"=TRUE, "code"=1, "source"=""} ("error constant"), "source"=w436) -> (w434:errorcluster)
        n163 = Unbundle By Name(w440) -> ("Scale Module Config.Process Name"=w443:string)
        n164 = Concatenate Strings(w443, "Invalid Message Recieved" ("text"), w435) -> (w441:string)
        n165 = call "Write to Log File.vi"("error in"=w434, "text"=w441) -> ()  [unwired: 9 in, 1 out]
      }
    }
    n166 = call "Error Handler - Message Handling Loop.vi"("error in (no error)"=w79, "Message Queue"=w77) -> ("dup error in"=w78:errorcluster, "dup Message Queue"=w65:refnum<queue>)  [unwired: 8 in]
  }
  n167 = while {
    tunnel: w21 -> [w457]
    tunnel: [w459] -> w27
    shift-right: [w458] -> w22
    shift-left: w25 -> [w463]
    tunnel: [w456] -> w15
    tunnel: w14 -> [w456]
    tunnel: w11 -> [w455]
    shift-right: [w452] -> _
    shift-left: w5 -> [w451]
    tunnel: [w447] -> w4
    tunnel: [w446] -> w3
    tunnel: w1 -> [w445]
    stop <- w462 stop-if-true
    # "Event Handling Loop"
    n168 = call "Dequeue Message.vi"("timeout in ms (-1)"=50, "Message Queue"=w455) -> ("error out"=w448:errorcluster, "Message Data"=w453:variant, "Message"=w454:string, "dup Message Queue"=w449:refnum<queue>)  [unwired: 6 in]
    n169 = Flush Queue(queue=w449, error in (no error)=w448) -> (queue out=w446:refnum<queue>)  [unwired: 2 out]
    n170 = case "Display Update" shown="\"Update\"" w454 {
      tunnel: w453 -> [_ w472]
      tunnel: [w464 w470] -> w452
      tunnel: w451 -> [w464 _]
      frame "False", Default {
      }
      frame "Update" {
        w469 = T10 {"Scale Value"=0.0, "Cycle Period"=500.0}  # SM Display
        n171 = Variant To Data(type=w469, Variant=w472) -> (data=w471:T10)  [unwired: 1 in, 1 out]
        n172 = Unbundle By Name(w471) -> ("Scale Value"=w467:dbl, "Cycle Period"=w470:dbl)
        n173 = property on="User Name" class="Str"() -> ("Value"=w465:string)  [unwired: 2 in, 2 out]
        n174 = Bundle By Name(cluster=cluster{"User Name":string, "g":dbl} {"User Name"="", "g"=0.0} ("Display Cluster"), "User Name"=w465, "g"=w467) -> (→"Display Cluster":cluster{"User Name":string, "g":dbl})
      }
    }
    n175 = event shown="[1] Panel Resize" {
      selector: w463 -> [_ _ _ _ _ _ _]
      dyn-events: [_ _ _ _ _ _ _] -> w458
      timeout: w452 -> [_ _ _ _ _ _ _]
      tunnel: [_ _ _ TRUE ("Discard?") TRUE ("Discard?") _ _] -> w462
      tunnel: w457 -> [w473 w481 w489 w497 w502 w508 w521]
      tunnel: [_ _ w487 w494 _ w510 _] -> w460
      tunnel: [w473 w481 w488 w500 w502 w509 w521] -> w461
      tunnel: w445 -> [_ _ _ w493 _ w505 _]
      event Timeout {
        n176 = event-data() -> ()  [unwired: 1 in, 1 out]
      }
      event Panel Resize {
        n177 = event-data() -> ("NewBnds"=w476:T11)  [unwired: 1 in]
        n178 = local read "Original Width"() -> (w480:u32)
        n179 = call "Front End Resize.vi"("Starting Font"=15.0, "Area to Font Division"=400.0, "Original Text Box Width"=76, "NewBnds"=w476, "Original Panel Width"=w480) -> ("New Text Box Width"=w475:u64, "New Font Size"=w474:dbl)  [unwired: 5 in]
        n180 = flat-sequence {
          tunnel: w474 -> [w485]
          tunnel: w475 -> [w484]
          tunnel: [w484] -> _
          frame #0 {
            n181 = property on="User Name" class="Str"("Text.Width"=w484) -> ()  [unwired: 2 in, 2 out]
            n182 = Multiply(x=w484, y=0.6) -> (x*y=w483:dbl)
            n183 = property on="User Name" class="Str"("Text.Height"=w483) -> ()  [unwired: 2 in, 2 out]
            n184 = property on="User Name" class="Str"("Text.FontSize"=w485) -> ()  [unwired: 2 in, 2 out]
          }
          frame #1 {
            n185 = property on="User Name" class="Str"("Text.SizeToText"=TRUE ("Text.Size to Text?")) -> ()  [unwired: 2 in, 2 out]
          }
        }
        n186 = property on="g" class="DigNum (strict)"("Label.FontSize"=w474) -> ()  [unwired: 2 in, 2 out]
        n187 = property on="g" class="DigNum (strict)"("NumText.FontSize"=w474) -> ()  [unwired: 2 in, 2 out]
        n188 = property on="g" class="DigNum (strict)"("Text Width"=w475) -> ()  [unwired: 2 in, 2 out]
      }
      event Panel Close? {
        w490 = TRUE  # Priority Message
        n189 = event-data() -> ()  [unwired: 1 in, 1 out]
        n190 = call-poly "Enqueue Message.vi"("Priority Message? (F)"=w490, "Message"="Confirm Quit", "Message Queue"=w489) -> ("error out"=w487:errorcluster, "dup Message Queue"=w488:refnum<queue>)  [unwired: 7 in]
        n191 = event-data("Discard?"=TRUE) -> ()  [unwired: 1 in, 1 out]
      }
      event "Exit": Value Change {
        w498 = TRUE  # Priority Message
        # "The UI Message Loop handles sending the Exit message to other loops."
        n192 = event-data() -> ()  [unwired: 1 in, 1 out]
        n193 = call-poly "Enqueue Message.vi"("Priority Message? (F)"=w498, "Message"="Exit", "Message Queue"=w497) -> ("error out"=w495:errorcluster, "dup Message Queue"=w500:refnum<queue>)  [unwired: 7 in]
        n194 = call "Generate Temporary Report.vi"("error in (no error)"=w495, "Line of Events"=string[] ["Exit Clicked"], "Module Name"=w493) -> ("error out"=w494:errorcluster)  [unwired: 8 in]
      }
      event User Event {
        # "The Message Handling Loop processed an \"Exit\" message, which fired this event to stop the Event Handling Loop."
        n195 = event-data() -> ()  [unwired: 1 in, 1 out]
        n196 = local write "Status"("Exit" ("Exit String")) -> ()
      }
      event "Settings Button": Mouse Down {
        # "Allow debugging during run with a ctrl click"
        n197 = event-data() -> ("PlatMods"=w507:T12)  [unwired: 1 in]
        n198 = Unbundle By Name(w507) -> ("Ctrl"=w506:bool)
        n199 = case shown="False" w506 {
          tunnel: [w512 w518] -> w510
          tunnel: [w517 w519] -> w509
          tunnel: w508 -> [w516 w519]
          tunnel: w505 -> [w511 _]
          frame False {
            n200 = call-poly "Enqueue Message.vi"("Message"="Launch Settings Dialog", "Message Queue"=w516) -> ("error out"=w513:errorcluster, "dup Message Queue"=w517:refnum<queue>)  [unwired: 8 in]
            n201 = call "Generate Temporary Report.vi"("error in (no error)"=w513, "Line of Events"=string[] ["Settings Dialog Opened"], "Module Name"=w511) -> ("error out"=w512:errorcluster)  [unwired: 8 in]
          }
          frame True {
            n202 = property class="VI"("BDWin.Open"=TRUE ("Block Diagram Window:Open")) -> (error out=w518:errorcluster)  [unwired: 2 in, 1 out]
          }
        }
      }
      event Key Down {
        n203 = event-data() -> ("ScanCode"=→"ScanCode":i16)  [unwired: 1 in]
      }
    }
    n204 = call "Error Handler - Event Handling Loop.vi"("error in (no error)"=w460, "Message Queue"=w461) -> ("dup error in"=w459:errorcluster, "dup Message Queue"=w447:refnum<queue>)  [unwired: 8 in]
  }
  n205 = call "Main Loop.vi"("error in (no error)"=w10, "Chart Notifier"=w16, "Message Queues"=w9) -> ("error out"=w17:errorcluster)  [unwired: 8 in]
  n206 = Unregister For Events(event registration refnum=w22, error in=w27) -> (error out=w23:errorcluster)
  n207 = Close Reference(reference=w15) -> ()  [unwired: 1 in, 1 out]
  n208 = Merge Errors(w23, w28, w10, w17) -> (w26:errorcluster)
  n209 = Release Queue(queue=w4) -> ()  [unwired: 2 in, 3 out]
  n210 = Release Queue(queue=w3) -> ()  [unwired: 2 in, 3 out]
  n211 = Release Queue(queue=w2) -> ()  [unwired: 2 in, 3 out]
  n212 = call "Destroy User Event - Stop.vi"("error in (no error)"=w26, "User Event - Stop"=w24) -> ("error out"=w6:errorcluster)  [unwired: 9 in]
  n213 = flat-sequence {
    tunnel: w6 -> [_]
    frame #0 {
      n214 = invoke class="VI" method="FP.Close"() -> ()  [unwired: 3 in, 3 out]
    }
  }
